vi "Superimpose Measurement Annotation.vi"(5 "Point A Image":refnum<class "Vec3d.lvclass">, 7 "Point B Image":refnum<class "Vec3d.lvclass">, 8 "error in":errorcluster, 9 "Point B":refnum<class "Vec3d.lvclass">, 10 "Point A":refnum<class "Vec3d.lvclass">, 11 "Image In":T1) -> (0 "error out":errorcluster, 3 "Image Out":T1)   [LabVIEW 2023]
uses:
  <vilib>/vision/Image Controls.llb/IMAQ Image.ctl
  Vec3d Class/Vec3d.lvclass
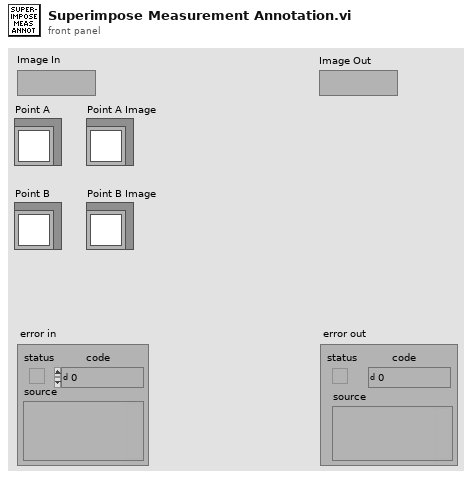
[diagram p1: front panel]
types:
  T1 = typedef "IMAQ Image.ctl" = refnum<image>
  T2 = cluster{"Left":i32, "Top":i32, "Right":i32, "Bottom":i32}
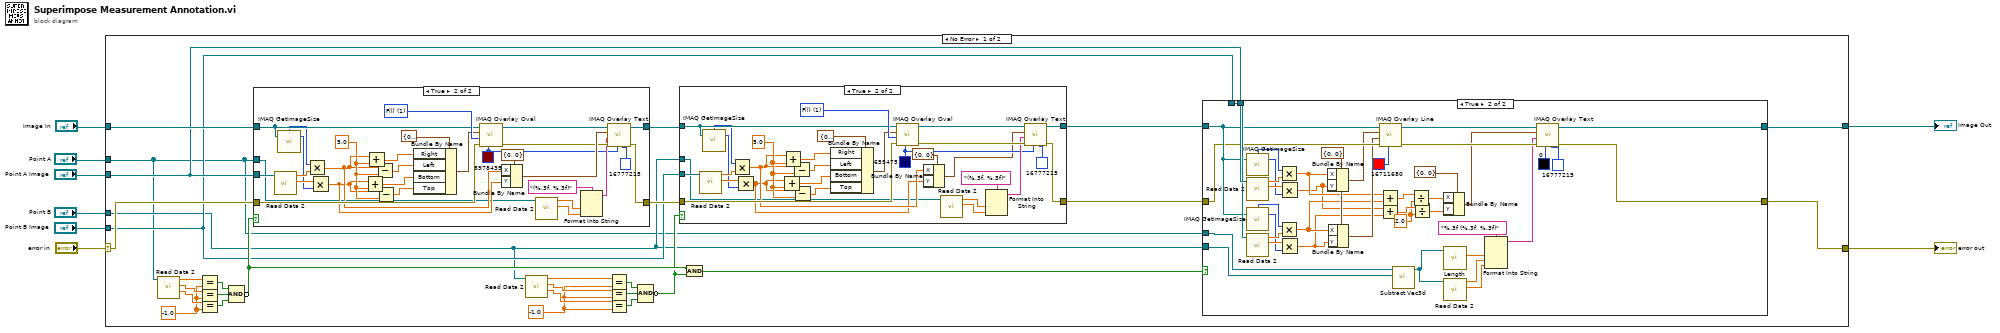
[diagram p0: block diagram]
diagram:
  n1 = case shown="No Error" "error in" {
    selector: "error in" -> [w22 w145]
    tunnel: "Image In" -> [w23 w146]
    tunnel: "Point A" -> [w9 _]
    tunnel: "Point A Image" -> [w14 _]
    tunnel: "Point B" -> [w10 _]
    tunnel: "Point B Image" -> [w11 _]
    tunnel: [w13 w146] -> w2
    tunnel: [w12 w145] -> w1
    frame No Error {
      w27 = -1.0 ("y")
      w34 = -1.0 ("y")
      n2 = call-dynamic "Read Data 2.vi"("Vec3d in"=w9) -> ("Z"=w35:dbl, "Y"=w36:dbl, "X"=w37:dbl)  [unwired: 7 in, 1 out]
      n3 = Equal?(x=w37, y=w34) -> (x = y?=w33:bool)
      n4 = Equal?(x=w36, y=w34) -> (x = y?=w32:bool)
      n5 = Equal?(x=w35, y=w34) -> (x = y?=w31:bool)
      n6 = Compound Arithmetic op=AND(w33, w32, w31) -> (invert w19:bool)
      n7 = case shown="True" w19 {
        tunnel: w9 -> [_ w121]
        tunnel: w14 -> [_ w142]
        tunnel: w23 -> [w114 w135]
        tunnel: [w114 w129] -> w21
        tunnel: w22 -> [w113 w144]
        tunnel: [w113 w122] -> w20
        frame False {
        }
        frame True {
          w141 = 5.0
          w115 = u32 8978435 ("Color")
          w143 = u32 1 items=["Frame", "Fill"] ("Drawing Mode (Frame)")
          n8 = call-dynamic "Read Data 2.vi"("Vec3d in"=w142) -> ("Y"=w132:dbl, "X"=w134:dbl)  [unwired: 7 in, 2 out]
          n9 = call "IMAQ GetImageSize"("Image"=w135) -> ("Y Resolution"=w131:i32, "X Resolution"=w133:i32)  [unwired: 3 in, 1 out]
          n10 = Multiply(x=w133, y=w134) -> (x*y=w126:dbl)
          n11 = Multiply(x=w132, y=w131) -> (x*y=w125:dbl)
          n12 = Add(x=w125, y=w141) -> (x+y=w137:dbl)
          n13 = Add(x=w126, y=w141) -> (x+y=w139:dbl)
          n14 = Subtract(x=w126, y=w141) -> (x-y=w138:dbl)
          n15 = Subtract(x=w125, y=w141) -> (x-y=w136:dbl)
          n16 = Bundle By Name(cluster=T2 {"Left"=0, "Top"=0, "Right"=0, "Bottom"=0} ("Bounding Rectangle"), "Right"=w139, "Left"=w138, "Bottom"=w137, "Top"=w136) -> (w128:T2)
          n17 = call "IMAQ Overlay Oval"("Color"=w115, "error in (no error)"=w144, "Drawing Mode (Frame)"=w143, "Bounding Rectangle"=w128, "Image"=w135) -> ("error out"=w123:errorcluster, "Image Out"=w130:T1)  [unwired: 5 in]
          n18 = Bundle By Name(cluster=cluster{"X":i32, "Y":i32} {"X"=0, "Y"=0} ("Origin"), "X"=w126, "Y"=w125) -> (w124:cluster{"X":i32, "Y":i32})
          n19 = call-dynamic "Read Data 2.vi"("Vec3d in"=w121) -> ("Y"=w118:dbl, "X"=w119:dbl)  [unwired: 7 in, 2 out]
          n20 = Format Into String(format string="(%.3f, %.3f)", w119, w118) -> (resulting string=w117:string)  [unwired: 2 in, 1 out]
          n21 = call "IMAQ Overlay Text"("BG Color (Transparent)"=u32 16777215, "Text Color (black)"=w115, "error in (no error)"=w123, "String"=w117, "Origin"=w124, "Image"=w130) -> ("error out"=w122:errorcluster, "Image Out"=w129:T1)  [unwired: 4 in]
        }
      }
      n22 = call-dynamic "Read Data 2.vi"("Vec3d in"=w10) -> ("Z"=w28:dbl, "Y"=w29:dbl, "X"=w30:dbl)  [unwired: 7 in, 1 out]
      n23 = Equal?(x=w30, y=w27) -> (x = y?=w26:bool)
      n24 = Equal?(x=w29, y=w27) -> (x = y?=w25:bool)
      n25 = Equal?(x=w28, y=w27) -> (x = y?=w24:bool)
      n26 = Compound Arithmetic op=AND(w26, w25, w24) -> (invert w18:bool)
      n27 = case shown="True" w18 {
        tunnel: w10 -> [_ w90]
        tunnel: w11 -> [_ w110]
        tunnel: w21 -> [w82 w103]
        tunnel: [w82 w97] -> w16
        tunnel: w20 -> [w81 w112]
        tunnel: [w81 w91] -> w15
        frame False {
        }
        frame True {
          w109 = 5.0
          w84 = u32 655475 ("Color")
          w111 = u32 1 items=["Frame", "Fill"] ("Drawing Mode (Frame)")
          n28 = call-dynamic "Read Data 2.vi"("Vec3d in"=w110) -> ("Y"=w100:dbl, "X"=w102:dbl)  [unwired: 7 in, 2 out]
          n29 = call "IMAQ GetImageSize"("Image"=w103) -> ("Y Resolution"=w99:i32, "X Resolution"=w101:i32)  [unwired: 3 in, 1 out]
          n30 = Multiply(x=w101, y=w102) -> (x*y=w94:dbl)
          n31 = Multiply(x=w100, y=w99) -> (x*y=w93:dbl)
          n32 = Add(x=w93, y=w109) -> (x+y=w105:dbl)
          n33 = Add(x=w94, y=w109) -> (x+y=w107:dbl)
          n34 = Subtract(x=w94, y=w109) -> (x-y=w106:dbl)
          n35 = Subtract(x=w93, y=w109) -> (x-y=w104:dbl)
          n36 = Bundle By Name(cluster=T2 {"Left"=0, "Top"=0, "Right"=0, "Bottom"=0} ("Bounding Rectangle"), "Right"=w107, "Left"=w106, "Bottom"=w105, "Top"=w104) -> (w96:T2)
          n37 = call "IMAQ Overlay Oval"("Color"=w84, "error in (no error)"=w112, "Drawing Mode (Frame)"=w111, "Bounding Rectangle"=w96, "Image"=w103) -> ("error out"=w92:errorcluster, "Image Out"=w98:T1)  [unwired: 5 in]
          n38 = Bundle By Name(cluster=cluster{"X":i32, "Y":i32} {"X"=0, "Y"=0} ("Origin"), "X"=w94, "Y"=w93) -> (w83:cluster{"X":i32, "Y":i32})
          n39 = call-dynamic "Read Data 2.vi"("Vec3d in"=w90) -> ("Y"=w87:dbl, "X"=w88:dbl)  [unwired: 7 in, 2 out]
          n40 = Format Into String(format string="(%.3f, %.3f)", w88, w87) -> (resulting string=w86:string)  [unwired: 2 in, 1 out]
          n41 = call "IMAQ Overlay Text"("BG Color (Transparent)"=u32 16777215, "Text Color (black)"=w84, "error in (no error)"=w92, "String"=w86, "Origin"=w83, "Image"=w98) -> ("error out"=w91:errorcluster, "Image Out"=w97:T1)  [unwired: 4 in]
        }
      }
      n42 = And(x=w19, y=w18) -> (x .and. y?=w17:bool)
      n43 = case shown="True" w17 {
        tunnel: w16 -> [w38 w70]
        tunnel: w15 -> [w39 w69]
        tunnel: w14 -> [_ w72]
        tunnel: w11 -> [_ w71]
        tunnel: [w38 w56] -> w13
        tunnel: [w39 w48] -> w12
        tunnel: w10 -> [_ w46]
        tunnel: w9 -> [_ w45]
        frame False {
        }
        frame True {
          w58 = 2.0 ("y")
          w67 = cluster{"X":i32, "Y":i32} {"X"=0, "Y"=0} ("Start Point")
          n44 = call "IMAQ GetImageSize"("Image"=w70) -> ("Y Resolution"=w77:i32, "X Resolution"=w79:i32)  [unwired: 3 in, 1 out]
          n45 = call-dynamic "Read Data 2.vi"("Vec3d in"=w72) -> ("Y"=w78:dbl, "X"=w80:dbl)  [unwired: 7 in, 2 out]
          n46 = call "IMAQ GetImageSize"("Image"=w70) -> ("Y Resolution"=w73:i32, "X Resolution"=w75:i32)  [unwired: 3 in, 1 out]
          n47 = call-dynamic "Read Data 2.vi"("Vec3d in"=w71) -> ("Y"=w74:dbl, "X"=w76:dbl)  [unwired: 7 in, 2 out]
          n48 = Multiply(x=w79, y=w80) -> (x*y=w64:dbl)
          n49 = Multiply(x=w75, y=w76) -> (x*y=w63:dbl)
          n50 = Multiply(x=w78, y=w77) -> (x*y=w62:dbl)
          n51 = Multiply(x=w74, y=w73) -> (x*y=w61:dbl)
          n52 = Bundle By Name(cluster=w67, "X"=w64, "Y"=w62) -> (w68:cluster{"X":i32, "Y":i32})
          n53 = Bundle By Name(cluster=w67, "X"=w63, "Y"=w61) -> (w66:cluster{"X":i32, "Y":i32})
          n54 = call "IMAQ Overlay Line"("Color"=u32 16711680, "error in (no error)"=w69, "End Point"=w66, "Start Point"=w68, "Image"=w70) -> ("error out"=w55:errorcluster, "Image Out"=w57:T1)  [unwired: 5 in]
          n55 = Add(x=w64, y=w63) -> (x+y=w60:dbl)
          n56 = Add(x=w62, y=w61) -> (x+y=w59:dbl)
          n57 = call "Subtract Vec3d.vi"("Vec3d in 2"=w46, "Vec3d in 1"=w45) -> ("Vec3d Class out"=w44:refnum<class "Vec3d.lvclass">)  [unwired: 8 in, 1 out]
          n58 = Divide(x=w60, y=w58) -> (x/y=w53:dbl)
          n59 = Divide(x=w59, y=w58) -> (x/y=w52:dbl)
          n60 = Bundle By Name(cluster=cluster{"X":i32, "Y":i32} {"X"=0, "Y"=0} ("Origin"), "X"=w53, "Y"=w52) -> (w51:cluster{"X":i32, "Y":i32})
          n61 = call-dynamic "Length.vi"("Vec3d in"=w44) -> ("Length"=w43:dbl)  [unwired: 8 in, 2 out]
          n62 = call-dynamic "Read Data 2.vi"("Vec3d in"=w44) -> ("Y"=w41:dbl, "X"=w42:dbl)  [unwired: 7 in, 2 out]
          n63 = Format Into String(format string="%.3f (%.3f, %.3f)", w43, w42, w41) -> (resulting string=w40:string)  [unwired: 2 in, 1 out]
          n64 = call "IMAQ Overlay Text"("BG Color (Transparent)"=u32 16777215, "Text Color (black)"=u32 0, "error in (no error)"=w55, "String"=w40, "Origin"=w51, "Image"=w57) -> ("error out"=w48:errorcluster, "Image Out"=w56:T1)  [unwired: 4 in]
        }
      }
    }
    frame Error {
    }
  }
  "Image Out" <- w2
  "error out" <- w1
